vi "dsf config session property name.vi"() -> (3 "confg session property name":string)   [LabVIEW 2020, in "DSF Shared.lvlib"]
uses:
  Shared/DSF Shared.lvlib
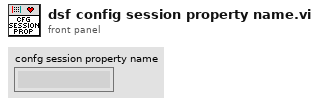
[diagram p1: front panel]
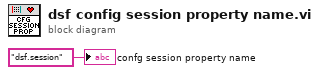
[diagram p0: block diagram]
diagram:
  "confg session property name" <- "dsf.session" ("Property Name")
